vi "convert.vi"(8 "error in (no error)":errorcluster, 9 "Codec":refnum<class "Codec.lvclass">, 10 "buffer":refnum<class "VideoFile.lvclass">, 11 "BitrateReader in":refnum<class "BitrateReader.lvclass">) -> (0 "error out":errorcluster, 2 "buffer out":refnum<class "VideoFile.lvclass">, 3 "BitrateReader out":refnum<class "BitrateReader.lvclass">)   [LabVIEW 2017, in "BitrateReader.lvclass"]
uses:
  BitrateReader.lvclass
  VideoFile Class/VideoFile.lvclass
  Codec Class/Codec.lvclass
  ConsoleOut/Print Options.ctl
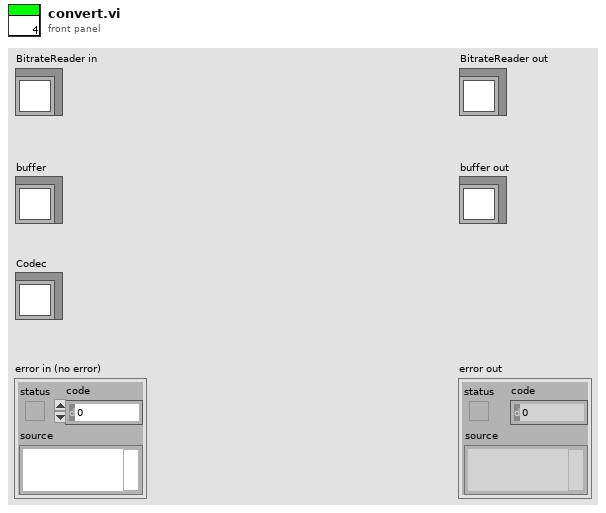
[diagram p1: front panel]
types:
  T1 = typedef "Print Options.ctl" = enum16{"Create", "Get Reference", "Print", "Print Header", "Close"}
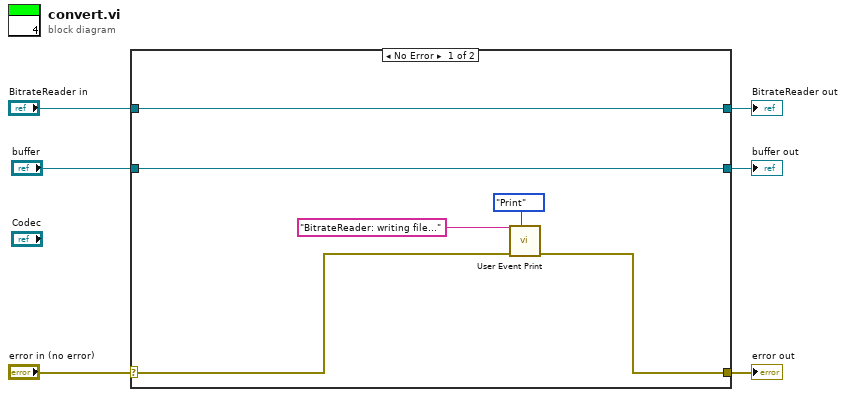
[diagram p0: block diagram]
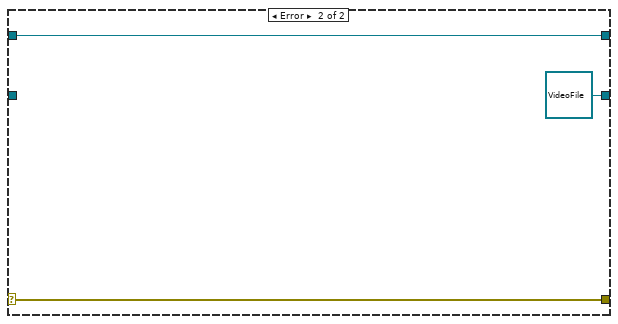
[diagram p2: hidden frame]
diagram:
  n1 = case shown="No Error" "error in (no error)" {
    selector: "error in (no error)" -> [w11 w15]
    tunnel: [w9 w15] -> w5
    tunnel: [w12 w14] -> w3
    tunnel: "BitrateReader in" -> [w12 w14]
    tunnel: "buffer" -> [w10 _]
    tunnel: [w10 refnum<class "VideoFile.lvclass"> refnum ("buffer")] -> w1
    frame No Error {
      n2 = call "User Event Print.vi"("Options"=Print_Options."Print", "error in (no error)"=w11, "String to Print"="BitrateReader: writing file...") -> ("error out"=w9:errorcluster)  [unwired: 7 in, 1 out]
    }
    frame Error {
    }
  }
  "error out" <- w5
  "BitrateReader out" <- w3
  "buffer out" <- w1
